vi "Read System Information.vi"(8 "error in (no error)":errorcluster, 11 "VISA resource name":refnum<visa-resource-name>) -> (0 "error out":errorcluster, 1 "Number of Ports":i32, 2 "Number of Traces":i32, 3 "VISA resource name out":refnum<visa-resource-name>, 4 "System Version":i32, 5 "Number of Channels":i32)   [LabVIEW 2020, in "Agilent ENA Series.lvlib"]
doc: "Reads system information."
uses:
  <instrlib>/Agilent ENA Series/Agilent ENA Series.lvlib
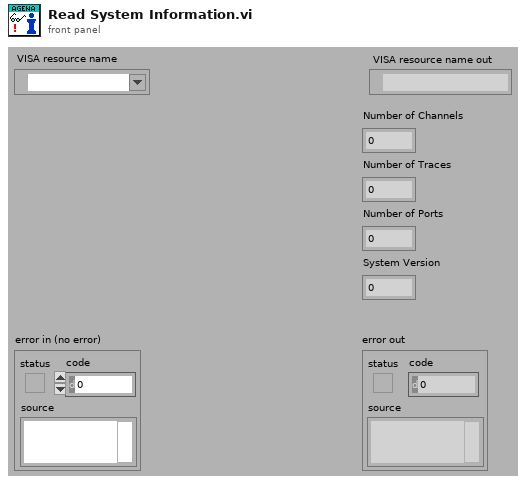
[diagram p1: front panel]
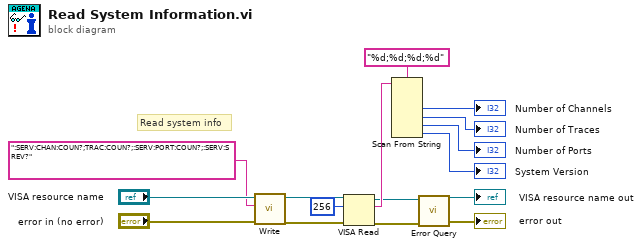
[diagram p0: block diagram]
diagram:
  # "Read system info"
  n1 = call <instrlib>:"Write.vi"("error in (no error)"="error in (no error)", "String ()"=":SERV:CHAN:COUN?;TRAC:COUN?;:SERV:PORT:COUN?;:SERV:SREV?" ("format string"), "VISA resource name"="VISA resource name") -> ("error out"=w14:errorcluster, "VISA resource name out"=w13:refnum<visa-resource-name>)  [unwired: 6 in, 1 out]
  n2 = VISA Read(VISA resource name=w13, byte count=u32 256, error in (no error)=w14) -> (VISA resource name out=w2:refnum<visa-resource-name>, read buffer=w11:string, error out=w3:errorcluster)  [unwired: 1 out]
  n3 = Scan From String(format string="%d;%d;%d;%d", input string=w11) -> (output 1=→"Number of Channels":i32, output 2=→"Number of Traces":i32, output 3=→"Number of Ports":i32, output 4=→"System Version":i32)  [unwired: 6 in, 3 out]
  n4 = call <instrlib>:"Error Query.vi"("error in (no error)"=w3, "VISA resource name"=w2) -> ("error out"=→"error out":errorcluster, "VISA resource name out"=→"VISA resource name out":refnum<visa-resource-name>)  [unwired: 6 in, 2 out]
